vi "DiagramDisable.vi"(8 "error in":errorcluster, 11 "reference":refnum<vi>) -> (0 "error out":errorcluster, 3 "DDS out":refnum<class "DiagramDisable.lvclass">)   [LabVIEW 2014, in "Raspberry Pi Compatible Compiler for LabVIEW.lvlib" / "DiagramDisable.lvclass"]
uses:
  DiagramDisable.lvclass
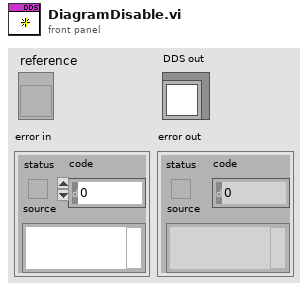
[diagram p1: front panel]
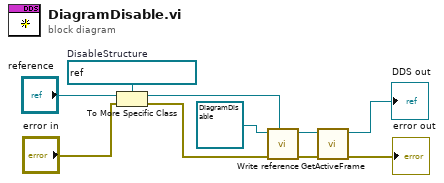
[diagram p0: block diagram]
diagram:
  w9 = refnum<vi> refnum  # DisableStructure
  n1 = To More Specific Class(target class=w9, reference="reference", error in="error in") -> (specific class reference=w6:refnum<vi>, error out=w7:errorcluster)
  n2 = call-dynamic "Write reference.vi"("reference"=w6, "error in"=w7, "GObject in"=refnum<class "DiagramDisable.lvclass"> refnum ("DDS In")) -> ("error out"=w3:errorcluster, "GObject out"=w4:refnum<class "DiagramDisable.lvclass">)  [unwired: 5 in]
  n3 = call-dynamic "GetActiveFrame.vi"("error in"=w3, "DiagramDisable in"=w4) -> ("error out"=→"error out":errorcluster, "DiagramDisable out"=→"DDS out":refnum<class "DiagramDisable.lvclass">)  [unwired: 6 in]
